vi "LED Test.vi"(0 "GEA2 Reference In":refnum<k24>, 11 "Error In":errorcluster) -> (4 "GEA2 Reference Out":refnum<k24>, 6 "Pass/Fail?":bool, 8 "Report Text":string, 15 "Error Out":errorcluster)   [LabVIEW 2016]
doc: "This VI performs the LED test. It first Writes the LED ERD to turn on all of the LEDs. Then prompts the user as to whether all LEDs are lit or not, for he Pass/Fail status."
uses:
  C:/Automation/DLLs/PC Dot Net/GeaCommunication.dll
  Common/LabVIEW GEA2 Toolkit/LabVIEW_GEA2_Toolkit.lvlibp/type defs/ERD Write Data In.ctl
  Common/LabVIEW GEA2 Toolkit/LabVIEW_GEA2_Toolkit.lvlibp/type defs/Data Type.ctl
  Common/LabVIEW GEA2 Toolkit/LabVIEW_GEA2_Toolkit.lvlibp/type defs/Source_Destination.ctl
  Common/LabVIEW GEA2 Toolkit/LabVIEW_GEA2_Toolkit.lvlibp
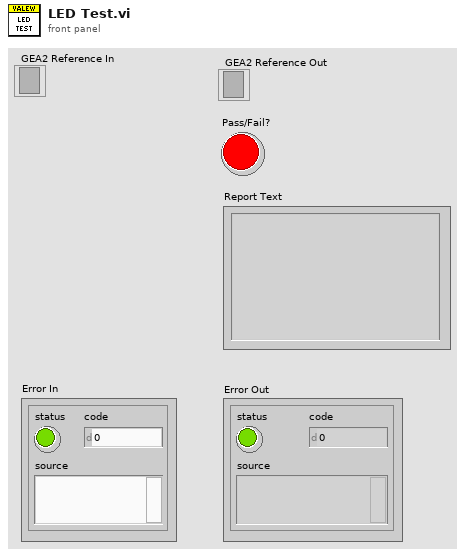
[diagram p1: front panel]
types:
  T1 = typedef "LabVIEW_GEA2_Toolkit.lvlibp/Source_Destination.ctl" = cluster{"Source":u8, "Destination":u8}
  T2 = typedef "LabVIEW_GEA2_Toolkit.lvlibp/ERD Write Data In.ctl" = cluster{"ERD Number":u16, "Data Type":T3, "Data":string}
  T3 = typedef "LabVIEW_GEA2_Toolkit.lvlibp/Data Type.ctl" = enum16{"string", "boolean", "uint8_t", "uint16_t", "uint32_t", "uint64_t", "int8_t", "int16_t", "int32_t", "int64_t"}
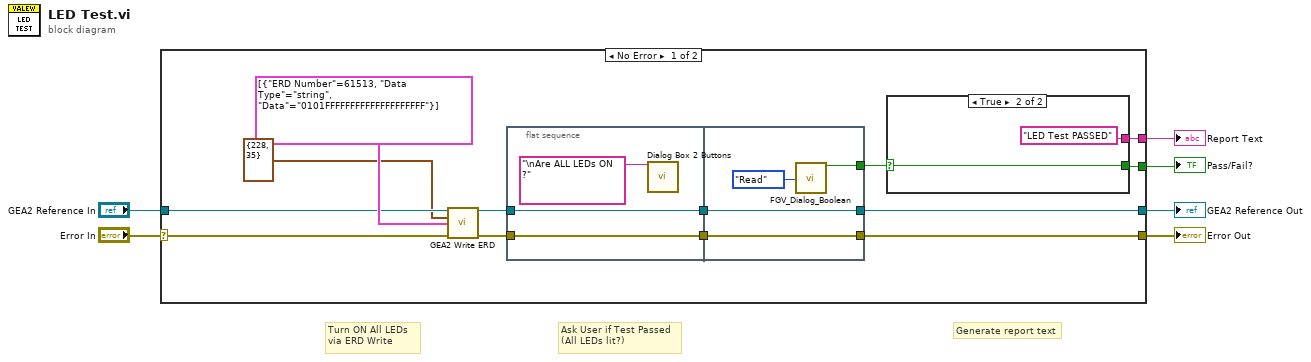
[diagram p0: block diagram]
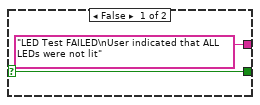
[diagram p2: hidden frame]
diagram:
  # "Generate report text"
  # "Ask User if Test Passed\n(All LEDs lit?)"
  # "Turn ON All LEDs\nvia ERD Write"
  n1 = case shown="No Error" "Error In" {
    selector: "Error In" -> [w10 w32]
    tunnel: "GEA2 Reference In" -> [w17 w31]
    tunnel: [w16 w32] -> w5
    tunnel: [w14 _] -> w4
    tunnel: [w13 _] -> w3
    tunnel: [w11 w31] -> w2
    frame No Error {
      n2 = call "GEA2 Write ERD.vi"("GEA2 Reference In"=w17, "GEA Inputs"=T1 {"Source"=228, "Destination"=35}, "Write ERD List"=T2[] [{"ERD Number"=61513, "Data Type"=enum."string", "Data"="0101FFFFFFFFFFFFFFFFFFFF"}], "Error In"=w10) -> ("GEA2 Reference Out"=w12:refnum<k24>, "Error Out"=w19:errorcluster)  [unwired: 9 in, 1 out]
      n3 = flat-sequence {
        tunnel: w19 -> [w26]
        tunnel: w12 -> [w25]
        tunnel: [w26] -> w9
        tunnel: [w25] -> w8
        tunnel: [w29] -> w11
        tunnel: [w30] -> w16
        tunnel: w9 -> [w30]
        tunnel: w8 -> [w29]
        tunnel: [w27] -> w7
        frame #0 {
          n4 = call "Dialog Box 2 Buttons.vi"("Input"="\nAre ALL LEDs ON ?" ("message")) -> ()  [unwired: 15 in]
        }
        frame #1 {
          n5 = call "FGV_Dialog_Boolean.vi"("Action"=enum16{"Write", "Read"}."Read") -> ("Boolean Out"=w27:bool)  [unwired: 13 in, 1 out]
        }
      }
      n6 = case shown="True" w7 {
        selector: w7 -> [w21 w23]
        tunnel: [w21 w23] -> w14
        tunnel: ["LED Test FAILED\nUser indicated that ALL LEDs were not lit" "LED Test PASSED"] -> w13
        frame False {
        }
        frame True {
        }
      }
    }
    frame Error {
    }
  }
  "Error Out" <- w5
  "Pass/Fail?" <- w4
  "Report Text" <- w3
  "GEA2 Reference Out" <- w2
